vi "FarFiledCapOneFrame.vi"   [LabVIEW 2018]
types:
  T1 = typedef "IMAQ Image.ctl" = refnum<image>
  T2 = cluster{"示波器":cluster{"Channel (0:Channel 1)":enum16{"Channel 1", "Channel 2", "Channel 3", "Channel 4"}, "电压范围":dbl, "触发电压":dbl, "时间范围":dbl, " 示波器VISA":refnum<visa-resource-name>, "时间范围 标签":u64, "电压范围 标签":u64, "触发电压 标签":u64}, "光谱仪":cluster{"SpecDataReference":refnum<queue>, "grating center":dbl, "Exposure Time (s)":dbl, "是否进行详细设置":bool, " 开始通信检查":bool, "通信成功？":bool, "波长":dbl}, " 近场相机":cluster{"曝光时间/100us":dbl, "模拟增益":i32, "控制套接字":i32, "IP 地址":string, " 采集套接字":i32, "  版本号":i32, "ImageData":T1, "  增益最大":i32, "  增益最小":i32, " 曝光最大":i32, " 曝光最小":i32, " 帧速":i32, " 同步切换":i32, "  曝光缩放":i32}, " 偏振仪":cluster{"电压范围":u64, "触发电压":u64, "时间范围":u64, "波长范围":enum16{"可见光 400-700nm", "近红外 700-1100nm"}, "可见光偏振测量仪VISA":refnum<visa-resource-name>, "近红外偏振测量仪VISA":refnum<visa-resource-name>}, " 功率计":cluster{"通道":enum16{"Channel 1", "Channel 2"}, "工作波长":u32, "单位":u64, "时间范围":u64, "IP地址":string, "端口":u32}, "能量计":cluster{"通道":enum16{"Channel 1", "Channel 2"}, "工作波长":u32, "单位":u64, "时间范围":u64, "IP地址":string, "端口":u32, "能量计量程":enum16{"200uJ", "20uJ", "2uJ", "200nJ"}}, "电机":cluster{"Channel (0:Channel 1)":enum16{"Channel 1", "Channel 2", "Channel 3", "Channel 4"}, "电压范围":u64, "触发电压":u64, "时间范围":u64}, " 远场相机":cluster{"曝光时间":i32, "模拟增益":i32, "控制套接字":i32, "IP 地址":string, " 采集套接字":i32, "  版本号":i32, "ImageData":T1, "  增益最大":i32, "  增益最小":i32, " 曝光最大":i32, " 曝光最小":i32, " 帧速":i32, " 同步切换":i32, "  曝光缩放":i32, "ImageData B":T1}}
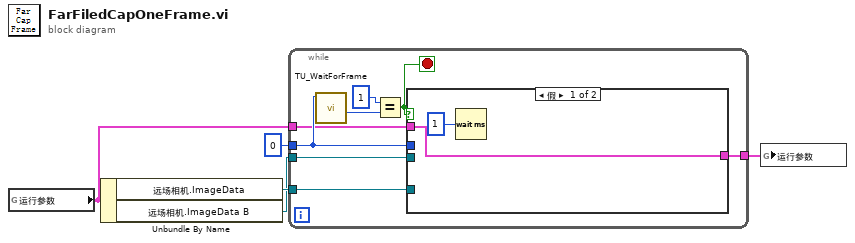
[diagram p0: block diagram]
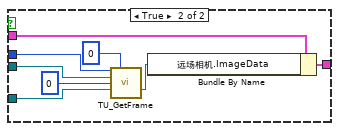
[diagram p2: hidden frame]
diagram:
  n1 = global read "参数.vi" "运行参数"() -> (w2:T2)
  n2 = Unbundle By Name(w2) -> ("远场相机.ImageData"=w4:T1, "远场相机.ImageData B"=w3:T1)
  n3 = while {
    tunnel: 0 -> [w10]
    tunnel: w4 -> [w9]
    tunnel: w3 -> [w8]
    tunnel: w2 -> [w7]
    tunnel: [w6] -> w1
    stop <- w11 stop-if-true
    n4 = call "TU_WaitForFrame.vi"("CameraIndex"=w10) -> ("Return Value"=w12:u32)  [unwired: 7 in, 1 out]
    n5 = Equal?(x=1, y=w12) -> (x = y?=w11:bool)
    n6 = case shown="假" w11 {
      tunnel: w10 -> [_ w21]
      tunnel: w9 -> [_ w20]
      tunnel: w8 -> [_ w19]
      tunnel: w7 -> [w14 w17]
      tunnel: [w14 w16] -> w6
      frame False {
        n7 = Wait (ms)(milliseconds to wait=u32 1 ("等待时间（毫秒）")) -> ()  [unwired: 1 out]
      }
      frame True {
        n8 = call "TU_GetFrame.vi"("CameraIndex"=w21, "nFuncSelect"=0, "ImageSRC_Average"=w19, "AverageCntIn"=0, "ImageSRC_Normal"=w20) -> ("Image_Normal"=w18:T1)  [unwired: 6 in, 4 out]
        n9 = Bundle By Name(cluster=w17, "远场相机.ImageData"=w18) -> (w16:T2)
      }
    }
  }
  n10 = global write "参数.vi" "运行参数"(w1) -> ()
